vi "Maximum Read.vi"(4 "error in (no error)":errorcluster, 6 "Container State":T3, 7 "Display State In":T1={"Window Handle"=refnum, "Maximum"=100, "State Change Action"=enum."Method - Initialize", "Running"=FALSE, "Visable Items"={"Label"=TRUE, "Caption"=FALSE}, "Value"=100, "Show Progress Bar"=FALSE}) -> (0 "error out":errorcluster, 2 "Value":u64, 3 "Display State Out":T1={"Window Handle"=refnum, "Maximum"=100, "State Change Action"=enum."Method - Initialize", "Running"=FALSE, "Visable Items"={"Label"=TRUE, "Caption"=FALSE}, "Value"=100, "Show Progress Bar"=FALSE})   [LabVIEW 2011, in "Taskbar Progress Bar.xctl"]
uses:
  Taskbar Progress Bar.xctl
  <vilib>/_xctls/Container State.ctl
  Abilities/TPB State.ctl
  TypeDefs/Dispaly State Change Methods.ctl
  <vilib>/_xctls/XControlSupport.lvlib
panel:
  # "Replace the Value Indicator below with an Indicator of desired type.\nDo not remove this Indicator or the others from the connector pane. \nDo not change the connector pane pattern.\nThe Value Indicator should always be the second terminal from top on the output side in the connector pane."
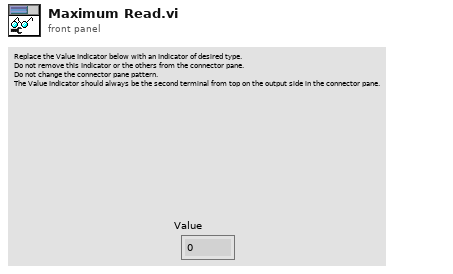
[diagram p1: front panel]
types:
  T1 = typedef "Taskbar Progress Bar.xctl/TPB State.ctl" = cluster{"Window Handle":refnum<k24>, "Maximum":u64, "State Change Action":T2, "Running":bool, "Visable Items":cluster{"Label":bool, "Caption":bool}, "Value":u64, "Show Progress Bar":bool}
  T2 = typedef "Taskbar Progress Bar.xctl/Dispaly State Change Methods.ctl" = enum16{"No Action", "Created", "Method - Initialize", "Method - Increment", "Method - Set Value", "Method - Pause", "Method - Error", "Method - Finish", "Property - Show Progress Bar"}
  T3 = typedef "XControlSupport.lvlib/Container State.ctl" = cluster{"Indicator?":bool, "Run Mode?":bool, " Refnum":refnum<vi>}
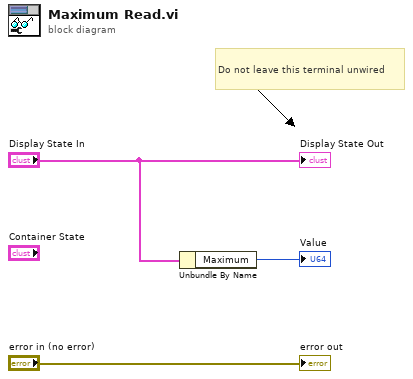
[diagram p0: block diagram]
diagram:
  # "Do not leave this terminal unwired"
  n1 = Unbundle By Name("Display State In") -> ("Maximum"=→"Value":u64)
  "error out" <- "error in (no error)"
  "Display State Out" <- "Display State In"
